vi "HotLotToExcel.vi"(8 "error in (no error)":errorcluster, 9 "Header":string, 10 "Input":string[][](array[string]), 11 "report in":refnum<class "NI_report.lvclass">) -> (0 "error out":errorcluster, 3 "report out":refnum<class "NI_report.lvclass">)   [LabVIEW 2012]
uses:
  <vilib>/Utility/NIReport.llb/NI_report.lvclass
  <vilib>/Utility/NIReport.llb/Append Text Table to Report (wrap).vi
  <vilib>/Utility/NIReport.llb/Excel/NI_Excel.lvclass
  <vilib>/addons/_office/NI_ReportGenerationToolkit.lvlib
panel:
  out "Row Headers":string[](array[string])
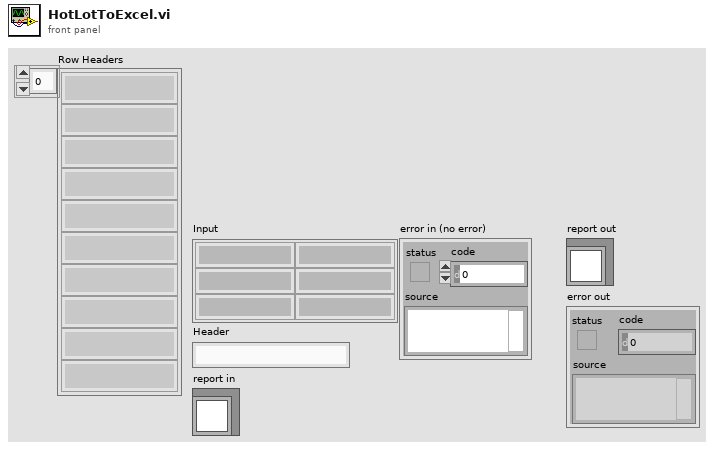
[diagram p1: front panel]
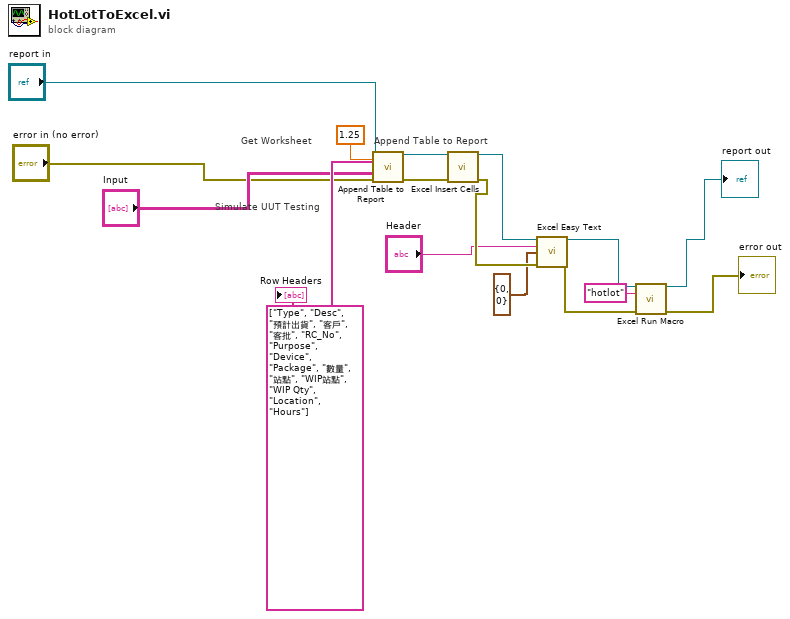
[diagram p0: block diagram]
diagram:
  w15 = string[] ["Type", "Desc", "預計出貨", "客戶", "客批", "RC_No", "Purpose", "Device", "Package", "數量", "站點", "WIP站點", "WIP Qty", "Location", "Hours"] ("row headers")
  # "Simulate UUT Testing"
  # "Append Table to Report"
  # "Get Worksheet"
  n1 = call-poly <vilib>:"Append Table to Report.vi"("report in"="report in", "column width (1)"=1.25, "column headers"=w15, "text data"="Input", "error in (no error)"="error in (no error)") -> ("report out"=w14:refnum<class "NI_report.lvclass">, "error out"=w13:errorcluster)  [unwired: 7 in, 2 out]
  n2 = call <vilib>:"Excel Insert Cells.vi"("report in"=w14, "error in (no error)"=w13) -> ("report out"=w12:refnum<class "NI_report.lvclass">, "error out"=w11:errorcluster)  [unwired: 12 in]
  n3 = call <vilib>:"Excel Easy Text.vi"("report in"=w12, "text"="Header", "start (-1, -1)"=cluster{"row":i32, "column":i32} {"row"=0, "column"=0} ("end (-1, -1)"), "error in (no error)"=w11) -> ("report out"=w4:refnum<class "NI_report.lvclass">, "error out"=w3:errorcluster)  [unwired: 7 in, 3 out]
  n4 = call <vilib>:"Excel Run Macro.vi"("report in"=w4, "macro name"="hotlot", "error in (no error)"=w3) -> ("report out"=→"report out":refnum<class "NI_report.lvclass">, "error out"=→"error out":errorcluster)  [unwired: 10 in, 1 out]
  "Row Headers" <- w15
